vi "Periodic Tasks.vi"(8 "error in":errorcluster) -> ()   [LabVIEW 2017]
doc: "This VI runs in parallel to other robot code. It can contain as many user-defined periodic loops as you need. These can carry out PID or other sorts of timed response."
uses:
  <vilib>/Rock Robotics/WPI/Joystick/WPI_JoystickDeviceEnum.ctl
  <vilib>/Rock Robotics/WPI/Ultrasonic/WPI_SonarMB1010AnalogDeviceRef.ctl
  <vilib>/Rock Robotics/WPI/AnalogChannel/WPI_AnalogChannelDevRef.ctl
  <vilib>/Rock Robotics/SystemInterfaces/AI/FPGA_AIChannel.ctl
  <vilib>/Rock Robotics/WPI/ThirdParty/Sensors/ADIS16448 IMU/ADI_IMU_ADIS16448_IMUDevRef.ctl
  <vilib>/Rock Robotics/SystemInterfaces/spilib/spi_bus.ctl
  <vilib>/Rock Robotics/WPI/Utilities/WPI_GetSetVariantRefNum.vi
  <vilib>/Rock Robotics/WPI/Ultrasonic/WPI_SonarMB1010AnalogRefNum Registry Get.vi
  Robot Global Data.vi
  <vilib>/Rock Robotics/WPI/Ultrasonic/WPI_SonarMB1010AnalogGetRange.vi
  <vilib>/Rock Robotics/WPI/ThirdParty/Sensors/ADIS16448 IMU/ADIS16448_IMU.lvlib
panel:
  out "Current Faults":bool[](array[boolean])
  out "Battery Voltage Fault":bool
  out "Temperature Fault":bool
  out "Hardware Fault":bool
  out "IMU Angles Out":T1
  out "Z Angle":dbl
  out "Sonar Distance":dbl
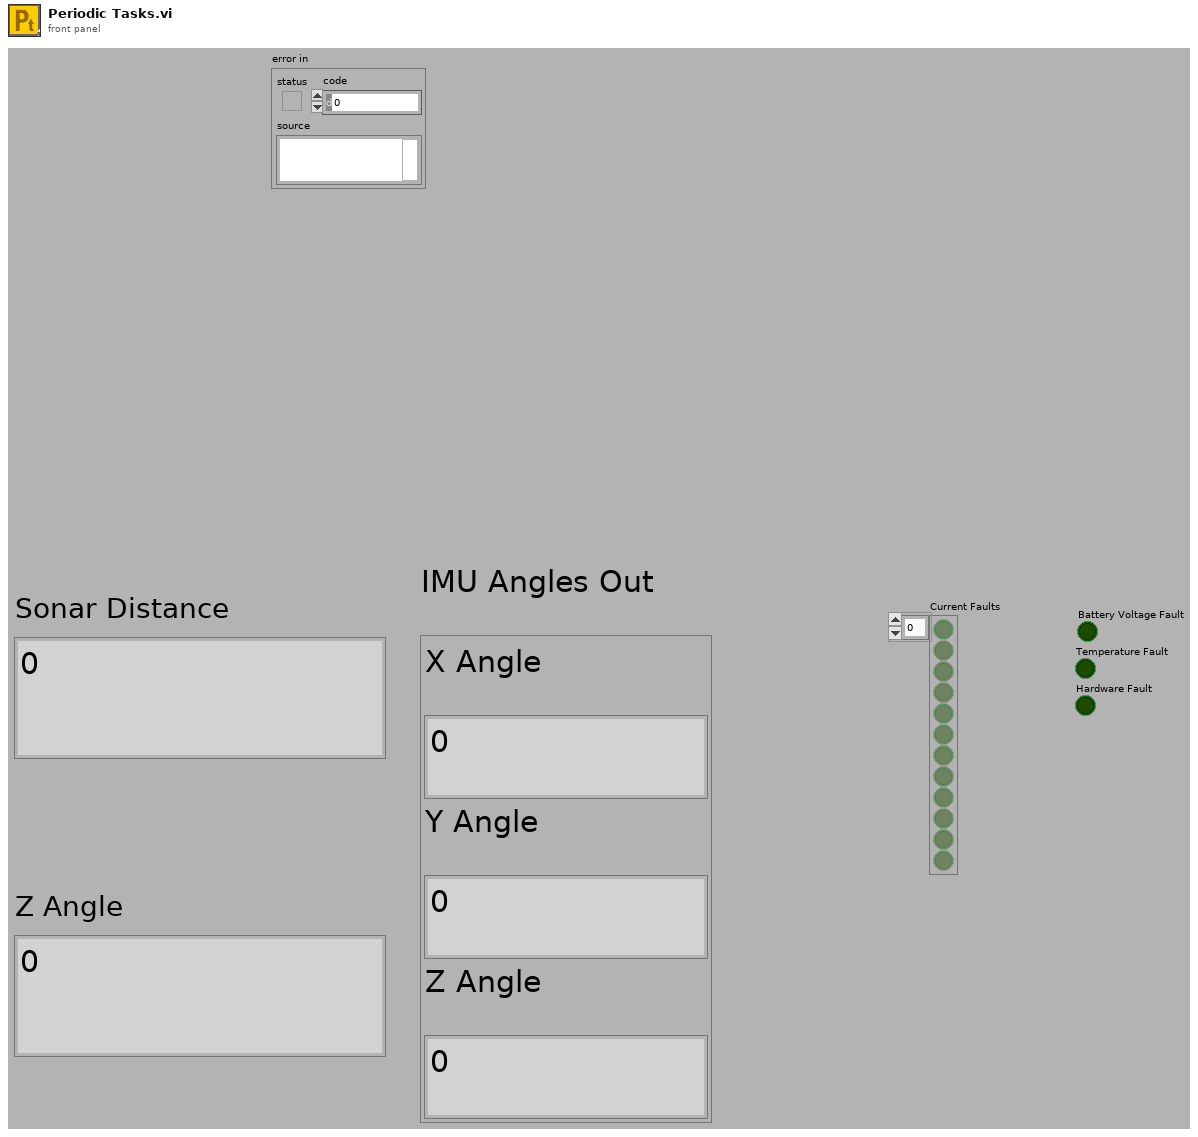
[diagram p1: front panel]
types:
  T1 = cluster{"X Angle":dbl, "Y Angle":dbl, "Z Angle":dbl}
  T2 = typedef "WPI_JoystickDeviceEnum.ctl" = enum16{"USB 0", "USB 1", "USB 2", "USB 3", "USB 4", "USB 5"}
  T3 = typedef "WPI_SonarMB1010AnalogDeviceRef.ctl" = cluster{"AIDeviceRef":T4, "Scaling factor (V/in)":dbl, "Average Bits":u8}
  T4 = typedef "WPI_AnalogChannelDevRef.ctl" = cluster{"DevStatus":errorcluster, "Analog Channel":T5}
  T5 = typedef "FPGA_AIChannel.ctl" = enum8{"AI 0", "AI 1", "AI 2", "AI 3", "AI MXP 0", "AI MXP 1", "AI MXP 2", "AI MXP 3", "Invalid"}
  T6 = typedef "ADIS16448_IMU.lvlib/ADI_IMU_ADIS16448_IMUDevRef.ctl" = cluster{"DevStatus":errorcluster, "Handle":i32, "SPI Bus":T7, "Device Found":bool, "Device Ready":bool, "Yaw Axis":enum16{"X", "Y", "Z"}, "AHRS Algorithm":enum16{"Complementary", "Madgwick"}, "Serial":u16, "Lot ID 2":u16, "Lot ID 1":u16, "Bytes Per Sample":u16, "Calibrate On Open?":bool}
  T7 = typedef "spi_bus.ctl" = enum16{"SPI On-Board, CS0", "SPI On-Board, CS1", "SPI On-Board, CS2", "SPI On-Board, CS3", "SPI MXP", "Invalid"}
  T8 = cluster{"Joystick 0":cluster{"Joystick 0":T2}, "Joystick 1":cluster{"Joystick 1":T2}, "Sonar":T3, "ADI IMU":T6}
  T9 = typedef "WPI_JoystickDevRef.ctl" = cluster{"Device":T2}
  T10 = typedef "WPI_DriverStationRobotMode2.ctl" = enum16{"Autonomous Disabled", "Autonomous Enabled", "Teleop Disabled", "Teleop Enabled", "Disconnected", "Finish", "Test Disabled", "Test Enabled", "Emergency Stopped"}
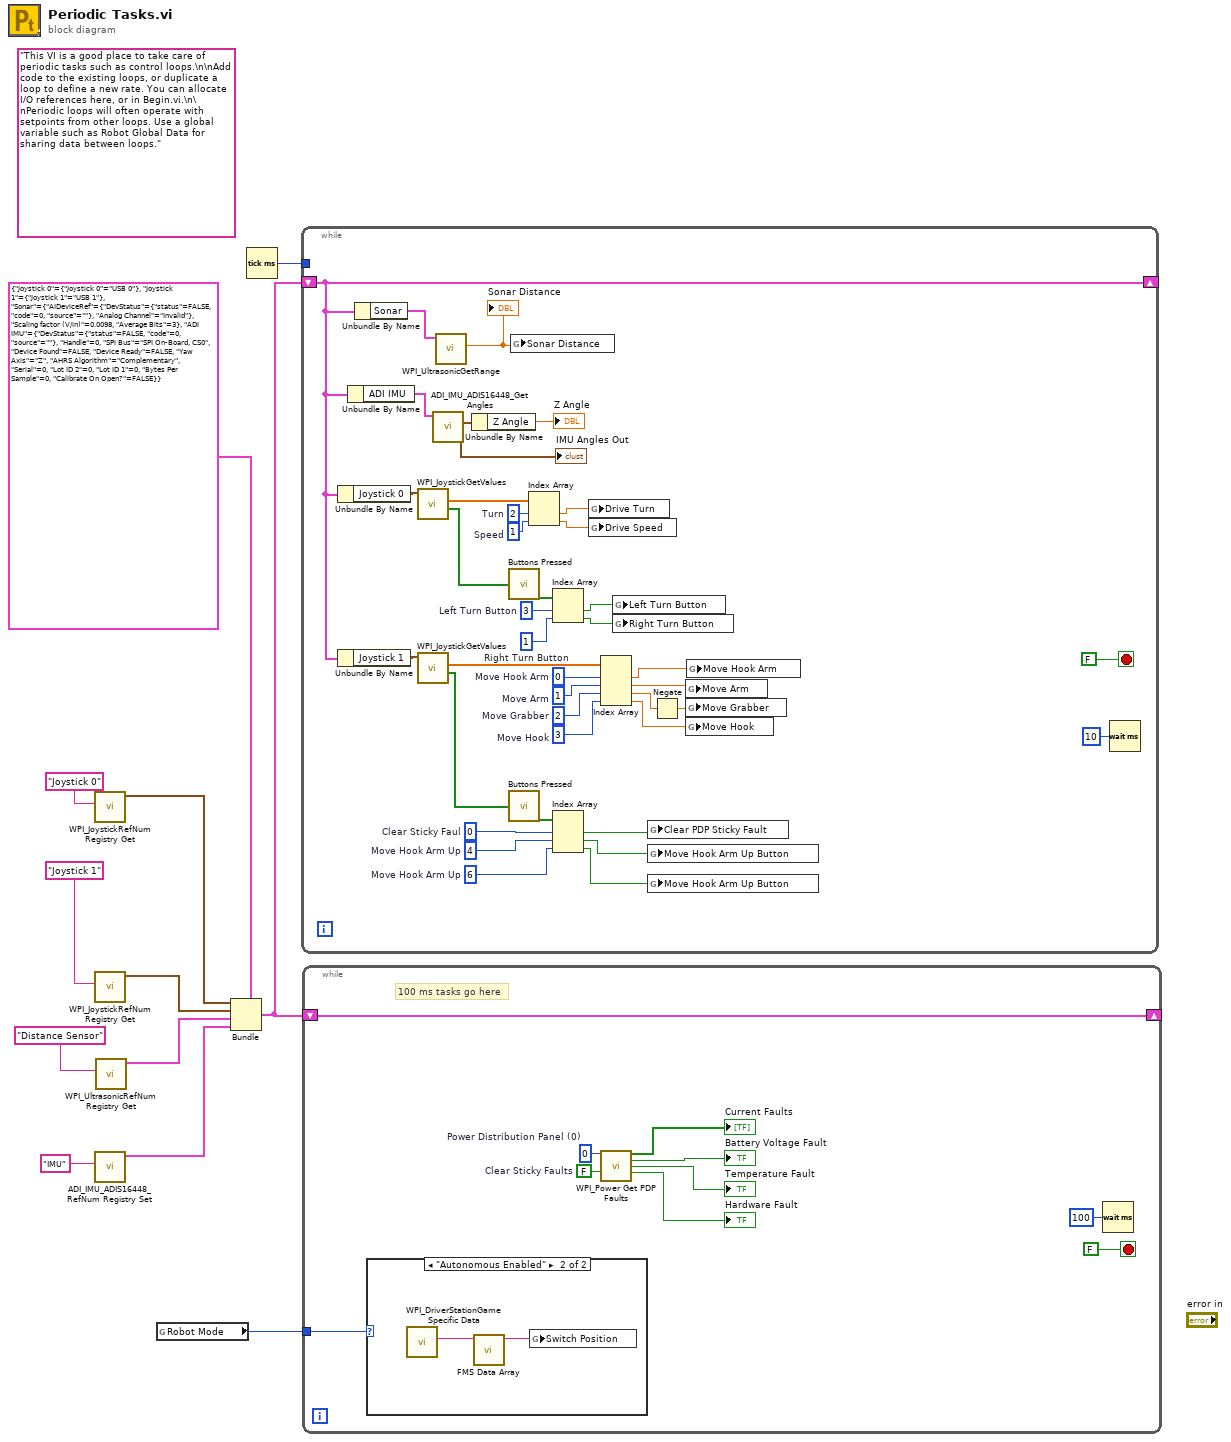
[diagram p0: block diagram]
diagram:
  (unwired) "This VI is a good place to take care of periodic tasks such as control loops.\n\nAdd code to the existing loops, or duplicate a loop to define a new rate. You can allocate I/O references here, or in Begin.vi.\n\nPeriodic loops will often operate with setpoints from other loops. Use a global variable such as Robot Global Data for sharing data between loops."
  n1 = call <vilib>:"WPI_JoystickRefNum Registry Get.vi"("refnum name"="Joystick 0") -> ("JoystickDevRef"=w9:T9)  [unwired: 1 in, 9 out]
  n2 = call <vilib>:"WPI_JoystickRefNum Registry Get.vi"("refnum name"="Joystick 1") -> ("JoystickDevRef"=w8:T9)  [unwired: 1 in, 9 out]
  n3 = call <vilib>:"ADI_IMU_ADIS16448_RefNum Registry Set.vi"("refnum name"="IMU") -> ("ADI IMU DevRef"=w2:T6)  [unwired: 9 in, 1 out]
  n4 = call-poly <vilib>:"WPI_UltrasonicRefNum Registry Get.vi"("refnum name"="Distance Sensor") -> ("SonarMB1010AnalogDevRef"=w3:T3)  [unwired: 9 in, 1 out]
  n5 = global read "Robot Global Data.vi" "Robot Mode"() -> (w1:T10)
  n6 = Bundle(cluster=T8 {"Joystick 0"={"Joystick 0"=enum."USB 0"}, "Joystick 1"={"Joystick 1"=enum."USB 1"}, "Sonar"={"AIDeviceRef"={"DevStatus"={"status"=FALSE, "code"=0, "source"=""}, "Analog Channel"=enum."Invalid"}, "Scaling factor (V/in)"=0.0098, "Average Bits"=3}, "ADI IMU"={"DevStatus"={"status"=FALSE, "code"=0, "source"=""}, "Handle"=0, "SPI Bus"=enum."SPI On-Board, CS0", "Device Found"=FALSE, "Device Ready"=FALSE, "Yaw Axis"=enum."Z", "AHRS Algorithm"=enum."Complementary", "Serial"=0, "Lot ID 2"=0, "Lot ID 1"=0, "Bytes Per Sample"=0, "Calibrate On Open?"=FALSE}}, "Joystick 0"=w9, "Joystick 1"=w8, "Sonar"=w3, "ADI IMU"=w2) -> (w7:T8)
  n7 = Tick Count (ms)() -> (millisecond timer value=w11:u32)
  n8 = while {
    shift-right: [w33] -> _
    shift-left: w7 -> [w33]
    tunnel: w11 -> [_]
    stop <- FALSE stop-if-true
    w14 = 6  # Move Hook Arm Up
    w16 = 4  # Move Hook Arm Up
    w27 = 3  # Move Hook
    w28 = 2  # Move Grabber
    w29 = 1  # Move Arm
    w30 = 0  # Move Hook Arm
    w31 = 1  # Speed
    w32 = 2  # Turn
    w37 = i8 0  # Clear Sticky Faul
    w42 = i8 1  # Right Turn Button
    w43 = i8 3  # Left Turn Button
    n9 = Unbundle By Name(w33) -> ("Joystick 0"=w39:cluster{"Joystick 0":T2})
    n10 = Unbundle By Name(w33) -> ("Joystick 1"=w38:cluster{"Joystick 1":T2})
    n11 = Unbundle By Name(w33) -> ("ADI IMU"=w40:T6)
    n12 = Unbundle By Name(w33) -> ("Sonar"=w41:T3)
    n13 = call <vilib>:"WPI_JoystickGetValues.vi"("JoystickDevRef"=w39) -> ("Buttons"=w45:bool[], "Axes"=w46:dbl[])  [unwired: 6 in, 3 out]
    n14 = call <vilib>:"WPI_JoystickGetValues.vi"("JoystickDevRef"=w38) -> ("Buttons"=w35:bool[], "Axes"=w34:dbl[])  [unwired: 6 in, 3 out]
    n15 = call <vilib>:"ADI_IMU_ADIS16448_Get Angles.vi"("ADI IMU DevRef"=w40) -> ("IMU Angles Out"=w48:T1)  [unwired: 7 in, 3 out]
    "IMU Angles Out" <- w48
    n16 = call-poly <vilib>:"WPI_UltrasonicGetRange.vi"("SonarMB1010AnalogDevRef"=w41) -> ("Distance"=w49:dbl)  [unwired: 8 in, 2 out]
    "Sonar Distance" <- w49
    n17 = Unbundle By Name(w48) -> ("Z Angle"=→"Z Angle":dbl)
    n18 = call "Buttons Pressed.vi"("Button Values"=w45) -> ("Button Presses"=w44:bool[])
    n19 = call "Buttons Pressed.vi"("Button Values"=w35) -> ("Button Presses"=w36:bool[])
    n20 = global write "Robot Global Data.vi" "Sonar Distance"(w49) -> ()
    n21 = Index Array(array=w46, index #1=w32, index #2=w31) -> (element #1=w23:dbl, element #2=w22:dbl)
    n22 = Index Array(array=w44, index #1=w43, index #2=w42) -> (element #1=w21:bool, element #2=w20:bool)
    n23 = Index Array(array=w36, index #1=w37, index #2=w16, index #3=w14) -> (element #1=w17:bool, element #2=w15:bool, element #3=w13:bool)
    n24 = global write "Robot Global Data.vi" "Drive Turn"(w23) -> ()
    n25 = global write "Robot Global Data.vi" "Drive Speed"(w22) -> ()
    n26 = Index Array(array=w34, index #1=w30, index #2=w29, index #3=w28, index #4=w27) -> (element #1=w18:dbl, element #2=w26:dbl, element #3=w25:dbl, element #4=w24:dbl)
    n27 = global write "Robot Global Data.vi" "Left Turn Button"(w21) -> ()
    n28 = global write "Robot Global Data.vi" "Right Turn Button"(w20) -> ()
    n29 = global write "Robot Global Data.vi" "Clear PDP Sticky Fault"(w17) -> ()
    n30 = global write "Robot Global Data.vi" "Move Hook Arm Up Button"(w15) -> ()
    n31 = global write "Robot Global Data.vi" "Move Hook Arm Up Button"(w13) -> ()
    n32 = Negate(x=w25) -> (-x=w19:dbl)
    n33 = global write "Robot Global Data.vi" "Move Arm"(w26) -> ()
    n34 = global write "Robot Global Data.vi" "Move Grabber"(w19) -> ()
    n35 = global write "Robot Global Data.vi" "Move Hook"(w24) -> ()
    n36 = global write "Robot Global Data.vi" "Move Hook Arm"(w18) -> ()
    n37 = Wait (ms)(milliseconds to wait=u32 10) -> ()  [unwired: 1 out]
  }
  n38 = while {
    shift-right: [w59] -> _
    shift-left: w7 -> [w59]
    tunnel: w1 -> [w52]
    stop <- FALSE stop-if-true
    w57 = FALSE  # Clear Sticky Faults
    w58 = u8 0  # Power Distribution Panel (0)
    # "100 ms tasks go here"
    n39 = case shown="\"Autonomous Enabled\"" w52 {
      frame Default {
      }
      frame "Autonomous Enabled" {
        n40 = call <vilib>:"WPI_DriverStationGame Specific Data.vi"() -> ("Game Specific Data"=w63:string)  [unwired: 11 in]
        n41 = call "FMS Data Array.vi"("Game Data"=w63) -> ("Switch"=w62:string)  [unwired: 8 in, 2 out]
        n42 = global write "Robot Global Data.vi" "Switch Position"(w62) -> ()
      }
    }
    n43 = call <vilib>:"WPI_Power Get PDP Faults.vi"("Power Distribution Panel (0)"=w58, "Clear Sticky Faults"=w57) -> ("Current Faults"=→"Current Faults":bool[], "Battery Voltage Fault"=→"Battery Voltage Fault":bool, "Temperature Fault"=→"Temperature Fault":bool, "Hardware Fault"=→"Hardware Fault":bool)  [unwired: 9 in, 1 out]
    n44 = Wait (ms)(milliseconds to wait=u32 100) -> ()  [unwired: 1 out]
  }
